vi "Get Power Sequence.vi"(11 "File Path":path) -> (1 "SMUs to Initialize (not in order)":T1[](array[typedef]), 2 "Power down Seq":T3[](array[typedef]) {"Power-down Seq" step=1; "Power-up Seq" step=1; "Wait Before Next (ms)" step=1; "Current Limit (A)" step=0.01 format="%.2g"; "Power-down Voltage (V)" step=0.01 format="%.2g"; "Power-up Voltage (V)" step=0.01 format="%.2g"}, 3 "Power up Seq":T3[](array[typedef]) {"Power-down Seq" step=1; "Power-up Seq" step=1; "Wait Before Next (ms)" step=1; "Current Limit (A)" step=0.01 format="%.2g"; "Power-down Voltage (V)" step=0.01 format="%.2g"; "Power-up Voltage (V)" step=0.01 format="%.2g"}, 5 "File Exists?":bool, 7 "Section Exists?":bool)   [LabVIEW 2023]
uses:
  DC Settings.ctl
  DC Ins Type.ctl
  DC Ins Initialize.ctl
  <vilib>/Utility/file.llb/Read Delimited Spreadsheet (string).vi
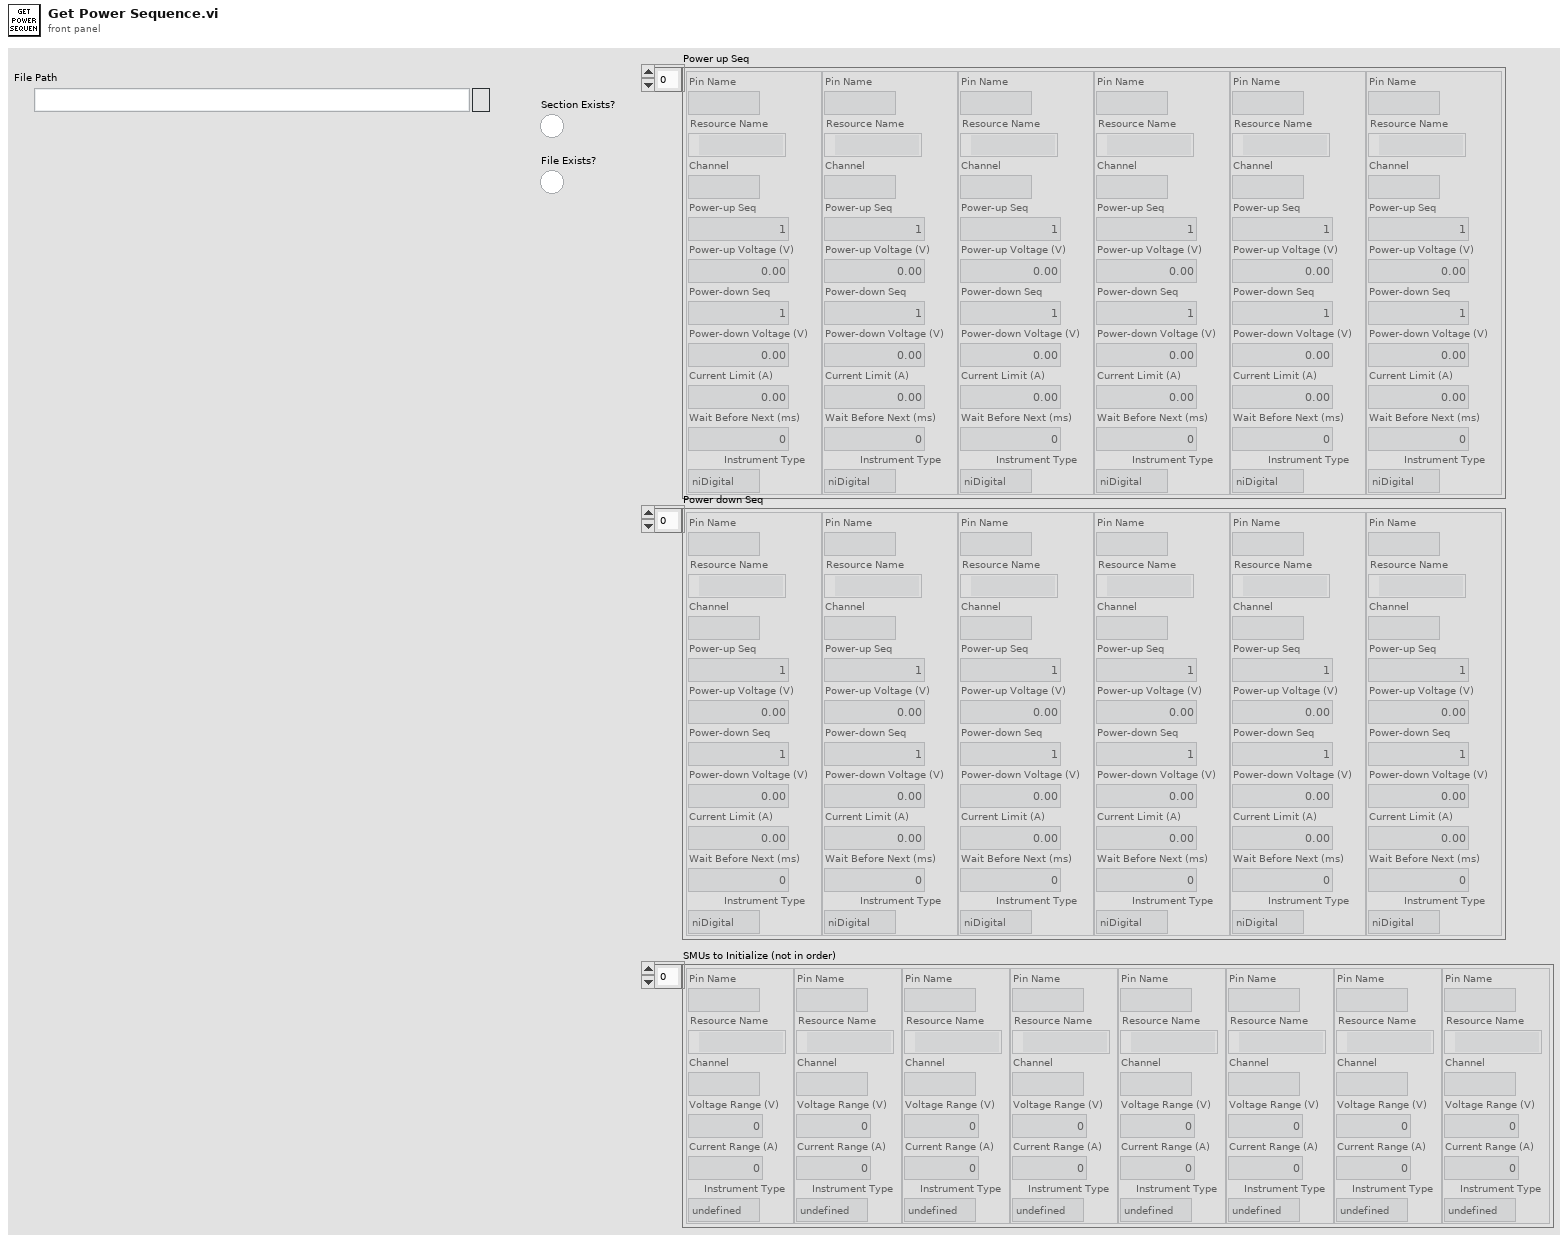
[diagram p1: front panel]
types:
  T1 = typedef "DC Ins Initialize.ctl" = cluster{"Pin Name":string, "Resource Name":refnum<k15>, "Channel":string, "Voltage Range (V)":dbl, "Current Range (A)":dbl, "Instrument Type":T2}
  T2 = typedef "DC Ins Type.ctl" = enum16{"niDigital", "niDCPower", "undefined"}
  T3 = typedef "DC Settings.ctl" = cluster{"Pin Name":string, "Resource Name":refnum<k15>, "Channel":string, "Power-up Seq":u32, "Power-up Voltage (V)":dbl, "Power-down Seq":u32, "Power-down Voltage (V)":dbl, "Current Limit (A)":dbl, "Wait Before Next (ms)":u32, "Instrument Type":T2}
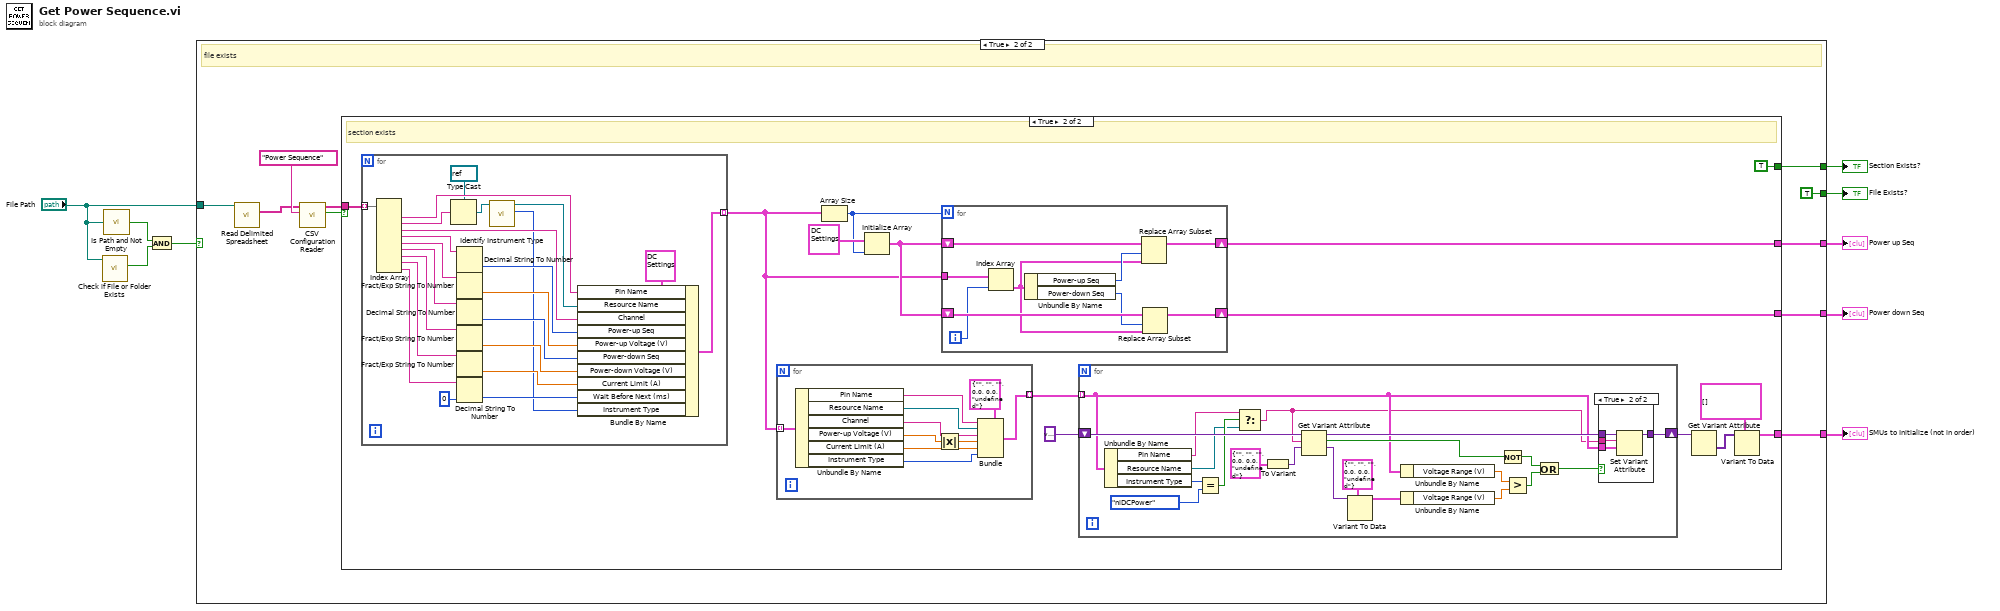
[diagram p0: block diagram]
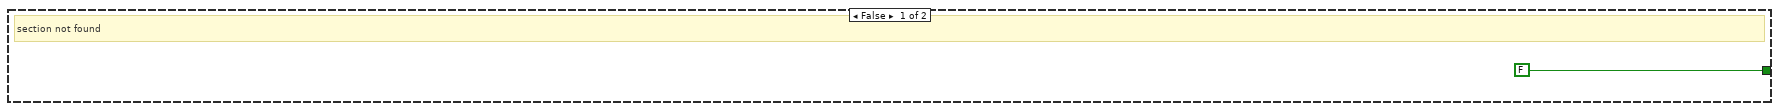
[diagram p3: hidden frame]
diagram:
  n1 = call <vilib>:"Check if File or Folder Exists.vi"("path"="File Path") -> ("file or folder exists?"=w3:bool)  [unwired: 8 in, 2 out]
  n2 = call <vilib>:"Is Path and Not Empty.vi"("path"="File Path") -> ("Is Path and Not Empty?"=w1:bool)  [unwired: 4 in]
  n3 = And(x=w1, y=w3) -> (x .and. y?=w4:bool)
  n4 = case shown="True" w4 {
    tunnel: "File Path" -> [_ w19]
    tunnel: [_ w18] -> w9
    tunnel: [_ w17] -> w8
    tunnel: [_ w16] -> w7
    tunnel: [_ TRUE] -> w6
    tunnel: [_ w10] -> w5
    frame False {
      # "file not found"
    }
    frame True {
      # "file exists"
      n5 = call-poly <vilib>:"Read Delimited Spreadsheet.vi"("file path (dialog if empty)"=w19) -> ("all rows"=w13:string[][])  [unwired: 9 in, 5 out]
      n6 = call "CSV Configuration Reader.vi"("Section"="Power Sequence" ("element"), "All CSV Configurations"=w13) -> ("Section Exists?"=w11:bool, "Extracted Configurations"=w12:string[][])  [unwired: 8 in]
      n7 = case shown="True" w11 {
        tunnel: [_ w30] -> w18
        tunnel: [_ w29] -> w17
        tunnel: [_ w26] -> w16
        tunnel: w12 -> [_ w25]
        tunnel: [FALSE TRUE] -> w10
        frame False {
          # "section not found"
        }
        frame True {
          # "section exists"
          n8 = for {
            tunnel: w25 -> [w83] mode=indexing
            tunnel: [w77] -> w31 mode=indexing
            n9 = Index Array(array=w83) -> (element #1=w67:string, element #2=w82:string, element #3=w66:string, element #4=w81:string, element #5=w72:string, element #6=w71:string, element #7=w73:string, element #8=w74:string, element #9=w75:string)  [unwired: 9 in]
            n10 = Type Cast(type=refnum<k15> refnum ("Resource Name"), x=w82) -> (*(type *) &x=w63:refnum<k15>)
            n11 = Decimal String To Number(string=w81) -> (number=w69:i32)  [unwired: 2 in, 1 out]
            n12 = Fract/Exp String To Number(string=w72) -> (number=w70:dbl)  [unwired: 3 in, 1 out]
            n13 = Decimal String To Number(string=w71) -> (number=w68:i32)  [unwired: 2 in, 1 out]
            n14 = Fract/Exp String To Number(string=w73) -> (number=w80:dbl)  [unwired: 3 in, 1 out]
            n15 = Fract/Exp String To Number(string=w74) -> (number=w79:dbl)  [unwired: 3 in, 1 out]
            n16 = Decimal String To Number(string=w75, default (0L)=u32 0 ("default (0 I32)")) -> (number=w78:u32)  [unwired: 1 in, 1 out]
            n17 = call "Identify Instrument Type.vi"("Resource Name in"=w63) -> ("Resource Type"=w61:T2, "Resource Name out"=w62:refnum<k15>)  [unwired: 9 in]
            n18 = Bundle By Name(cluster=T3 {"Pin Name"="", "Resource Name"="", "Channel"="", "Power-up Seq"=0, "Power-up Voltage (V)"=0.0, "Power-down Seq"=0, "Power-down Voltage (V)"=0.0, "Current Limit (A)"=0.0, "Wait Before Next (ms)"=0, "Instrument Type"=enum."niDigital"} ("Pin Config"), "Pin Name"=w67, "Resource Name"=w62, "Channel"=w66, "Power-up Seq"=w69, "Power-up Voltage (V)"=w70, "Power-down Seq"=w68, "Power-down Voltage (V)"=w80, "Current Limit (A)"=w79, "Wait Before Next (ms)"=w78, "Instrument Type"=w61) -> (w77:T3)
          }
          n19 = for {
            tunnel: w31 -> [w93] mode=indexing
            tunnel: [w89] -> w22 mode=indexing
            n20 = Unbundle By Name(w93) -> ("Pin Name"=w92:string, "Resource Name"=w91:refnum<k15>, "Channel"=w90:string, "Power-up Voltage (V)"=w87:dbl, "Current Limit (A)"=w86:dbl, "Instrument Type"=w84:T2)
            n21 = Absolute Value(x=w87) -> (abs(x)=w85:dbl)
            n22 = Bundle(cluster=T1 {"Pin Name"="", "Resource Name"="", "Channel"="", "Voltage Range (V)"=0.0, "Current Range (A)"=0.0, "Instrument Type"=enum."undefined"}, "Pin Name"=w92, "Resource Name"=w91, "Channel"=w90, "Voltage Range (V)"=w85, "Current Range (A)"=w86, "Instrument Type"=w84) -> (w89:T1)
          }
          n23 = Array Size(array=w31) -> (size(s)=w33:i32)
          n24 = Initialize Array(T3 {"Pin Name"="", "Resource Name"="", "Channel"="", "Power-up Seq"=0, "Power-up Voltage (V)"=0.0, "Power-down Seq"=0, "Power-down Voltage (V)"=0.0, "Current Limit (A)"=0.0, "Wait Before Next (ms)"=0, "Instrument Type"=enum."niDigital"} ("Pin Config"), w33) -> (w32:T3[])
          n25 = for {
            N: w33 -> [_]
            shift-right: [w99] -> w30
            shift-left: w32 -> [w101]
            tunnel: w31 -> [w102]
            shift-right: [w97] -> w29
            shift-left: w32 -> [w98]
            i -> [w94]
            n26 = Index Array(array=w102, index=w94) -> (element=w95:T3)
            n27 = Unbundle By Name(w95) -> ("Power-up Seq"=w100:u32, "Power-down Seq"=w96:u32)
            n28 = Replace Array Subset(array=w101, new element=w95, index=w100) -> (w99:T3[])
            n29 = Replace Array Subset(array=w98, new element=w95, index=w96) -> (w97:T3[])
          }
          n30 = for {
            tunnel: w22 -> [w41] mode=indexing
            shift-right: [w55] -> w23
            shift-left: variant -> [w54]
            n31 = Unbundle By Name(w41) -> ("Pin Name"=w37:string, "Resource Name"=w38:refnum<k15>, "Instrument Type"=w40:T2)
            n32 = Equal?(x=w40, y=DC_Ins_Type."niDCPower") -> (x = y?=w39:bool)
            n33 = Select(t=w37, s=w39, f=w38) -> (s? t:f=w36:string)
            n34 = To Variant(anything=T1 {"Pin Name"="", "Resource Name"="", "Channel"="", "Voltage Range (V)"=0.0, "Current Range (A)"=0.0, "Instrument Type"=enum."undefined"} ("Pin Config")) -> (Variant=w46:variant)
            n35 = Get Variant Attribute(Variant=w54, name=w36, default value (empty Variant)=w46) -> (duplicate Variant=w52:variant, found=w43:bool, value=w51:variant)  [unwired: 1 in, 1 out]
            n36 = Variant To Data(type=T1 {"Pin Name"="", "Resource Name"="", "Channel"="", "Voltage Range (V)"=0.0, "Current Range (A)"=0.0, "Instrument Type"=enum."undefined"} ("Pin Config"), Variant=w51) -> (data=w50:T1)  [unwired: 1 in, 1 out]
            n37 = Unbundle By Name(w41) -> ("Voltage Range (V)"=w49:dbl)
            n38 = Unbundle By Name(w50) -> ("Voltage Range (V)"=w48:dbl)
            n39 = Not(x=w43) -> (.not. x?=w42:bool)
            n40 = Greater?(x=w49, y=w48) -> (0:w44:bool)
            n41 = Or(x=w42, y=w44) -> (x .or. y?=w45:bool)
            n42 = case shown="True" w45 {
              tunnel: [w56 w60] -> w55
              tunnel: w36 -> [_ w59]
              tunnel: w52 -> [w56 w58]
              tunnel: w41 -> [_ w57]
              frame False {
              }
              frame True {
                n43 = Set Variant Attribute(Variant=w58, name=w59, value=w57) -> (Variant out=w60:variant)  [unwired: 1 in, 2 out]
              }
            }
          }
          n44 = Get Variant Attribute(Variant=w23) -> (values=w28:variant[])  [unwired: 3 in, 3 out]
          n45 = Variant To Data(type=T1[] [] ("Array"), Variant=w28) -> (data=w26:T1[])  [unwired: 1 in, 1 out]
        }
      }
    }
  }
  "Power up Seq" <- w9
  "Power down Seq" <- w8
  "SMUs to Initialize (not in order)" <- w7
  "File Exists?" <- w6
  "Section Exists?" <- w5
